vi "Write Key (U32).vi"(7 "section":string, 8 "error in (no error)":errorcluster, 9 "value":u32, 10 "key":string, 11 "refnum":T1) -> (0 "error out":errorcluster, 2 "found?":bool, 3 "refnum out":T1)   [LabVIEW 2020, in "NI_LVConfig.lvlib"]
doc: "Writes a value to a key in a specified section of the configuration data identified by <B>refnum</B>. This VI modifies data in memory. To write data to disk, use the Close Config Data VI. Wire data to the <B>value</B> input to determine the polymorphic instance to use or manually select the instance."
uses:
  NI_LVConfig.lvlib
  Config Data RefNum.ctl
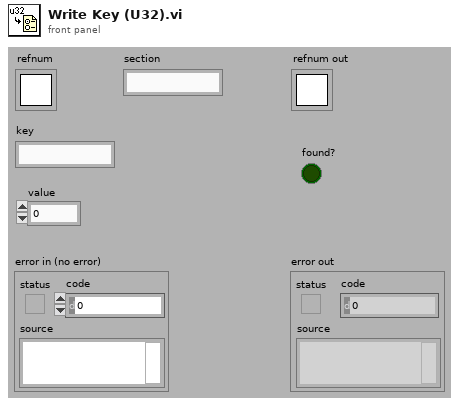
[diagram p1: front panel]
types:
  T1 = typedef "NI_LVConfig.lvlib/Config Data RefNum.ctl" = refnum<k1>
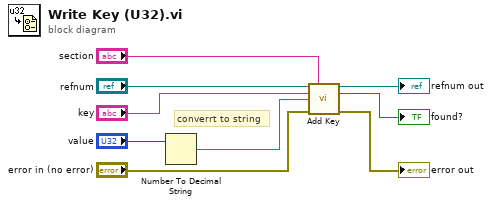
[diagram p0: block diagram]
diagram:
  # "converrt to string"
  n1 = Number To Decimal String(number="value") -> (decimal integer string=w3:string)  [unwired: 1 out]
  n2 = call "Add Key.vi"("refnum"="refnum", "section"="section", "key"="key", "value"=w3, "error in (no error)"="error in (no error)") -> ("refnum out"=→"refnum out":T1, "key exists?"=→"found?":bool, "error out"=→"error out":errorcluster)  [unwired: 2 in, 6 out]
